vi "TDT-Get Spikes.vi"(0 "Data":T1={"TTankX"=refnum, "TDevAccX"=refnum, "LastTime"=0.0, "error"={"status"=FALSE, "code"=0, "source"=""}, "Block Name"="", "Circuit Tag"="", "Tank Name"="", "NumTicks"=0, "LastTick"=0.0, "Idle?"=FALSE, "Wait (ms)"=1000, "LastArtf"=0.0, "LastTosc"=0.0}, 7 "Max Read":i32=1000, 11 "error in (no error)":errorcluster, 13 "Tetrode":bool) -> (4 "Got 'em all":bool, 8 "Spike times":dbl[][](array[numeric]), 14 "Last Time":dbl, 15 "error out":errorcluster)   [LabVIEW 2015]
uses:
  TDT Interface Data.ctl
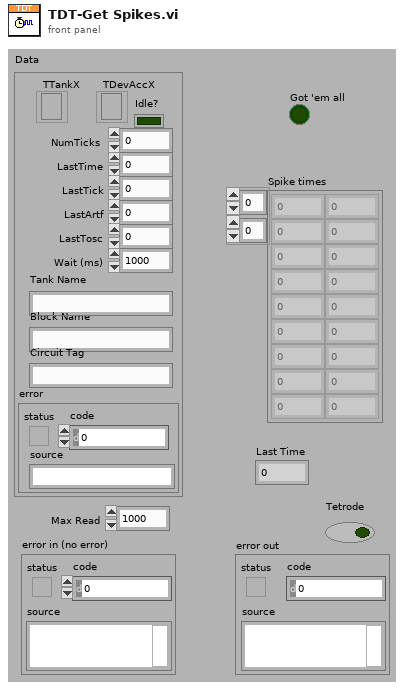
[diagram p1: front panel]
types:
  T1 = typedef "TDT Interface Data.ctl" = cluster{"TTankX":refnum<k7>, "TDevAccX":refnum<k7>, "LastTime":dbl, "error":errorcluster, "Block Name":string, "Circuit Tag":string, "Tank Name":string, "NumTicks":i32, "LastTick":dbl, "Idle?":bool, "Wait (ms)":u32, "LastArtf":dbl, "LastTosc":dbl}
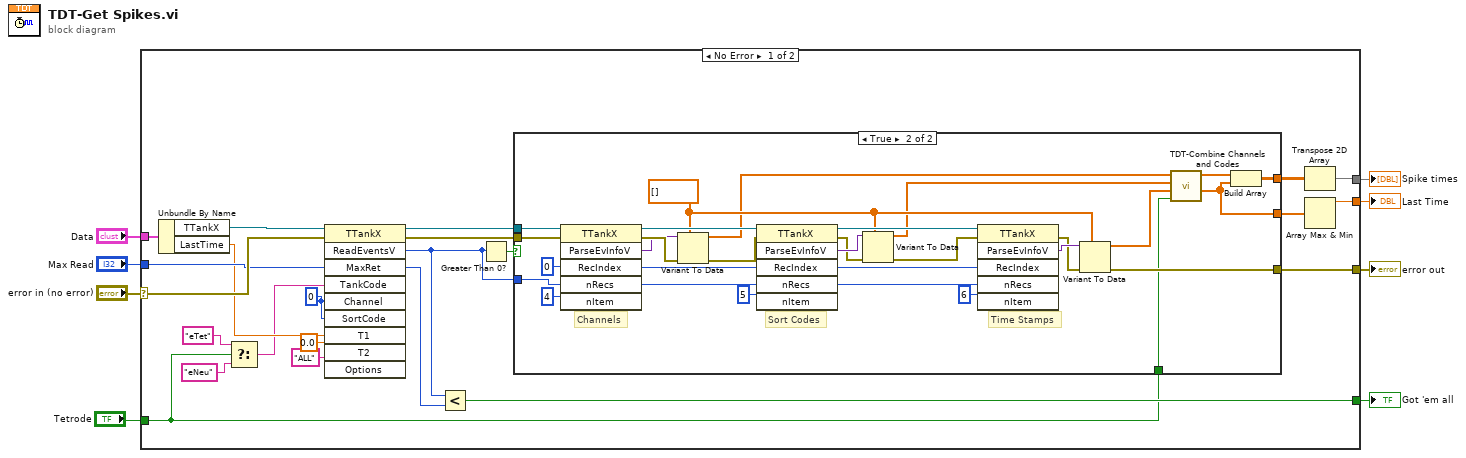
[diagram p0: block diagram]
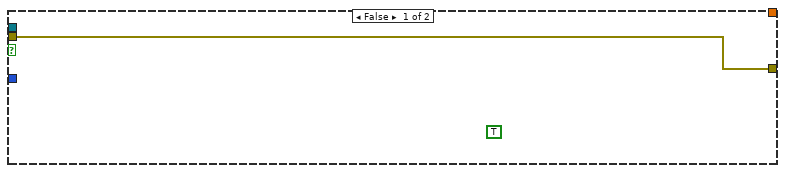
[diagram p2: hidden frame]
diagram:
  n1 = case shown="No Error" "error in (no error)" {
    selector: "error in (no error)" -> [w29 w63]
    tunnel: "Data" -> [w31 _]
    tunnel: "Max Read" -> [w28 _]
    tunnel: [w13 w63] -> w5
    tunnel: [w26 _] -> w4
    tunnel: [w15 _] -> w3
    tunnel: [w14 _] -> w2
    tunnel: "Tetrode" -> [w9 _]
    frame No Error {
      w22 = 0 ("Channel")
      n2 = Unbundle By Name(w31) -> ("TTankX"=w30:refnum<k7>, "LastTime"=w27:dbl)
      n3 = Select(t="eTet" ("TankCode"), s=w9, f="eNeu" ("TankCode")) -> (s? t:f=w10:string)
      n4 = invoke class="TTankX" method="ReadEventsV"(reference=w30, error in=w29, "MaxRet"=w28, "TankCode"=w10, "Channel"=w22, "SortCode"=w22, "T1"=w27, "T2"=0.0, "Options"="ALL") -> (reference out=w20:refnum<k7>, error out=w19:errorcluster, "ReadEventsV"=w17:i32, "MaxRet"=w21:i32)  [unwired: 1 in, 6 out]
      n5 = Less?(x=w17, y=w21) -> (x < y?=w14:bool)
      n6 = Greater Than 0?(x=w17) -> (x > 0?=w18:bool)
      n7 = case shown="True" w18 {
        tunnel: w20 -> [_ w62]
        tunnel: w19 -> [w32 w61]
        tunnel: w17 -> [_ w59]
        tunnel: [_ w36] -> w25
        tunnel: [w32 w54] -> w13
        tunnel: [_ w33] -> w16
        tunnel: w9 -> [_ w35]
        frame False {
          (unwired) TRUE
        }
        frame True {
          w41 = dbl[] []
          # "Time Stamps"
          # "Sort Codes"
          # "Channels"
          n8 = invoke class="TTankX" method="ParseEvInfoV"(reference=w62, error in=w61, "RecIndex"=0, "nRecs"=w59, "nItem"=4) -> (reference out=w51:refnum<k7>, error out=w57:errorcluster, "ParseEvInfoV"=w52:variant, "RecIndex"=w49:i32, "nRecs"=w48:i32)  [unwired: 1 in, 1 out]
          n9 = Variant To Data(error in=w57, type=w41, Variant=w52) -> (data=w39:dbl[], error out=w42:errorcluster)
          n10 = invoke class="TTankX" method="ParseEvInfoV"(reference=w51, error in=w42, "RecIndex"=w49, "nRecs"=w48, "nItem"=5) -> (reference out=w50:refnum<k7>, error out=w43:errorcluster, "ParseEvInfoV"=w44:variant, "RecIndex"=w45:i32, "nRecs"=w46:i32)  [unwired: 1 in, 1 out]
          n11 = Variant To Data(error in=w43, type=w41, Variant=w44) -> (data=w38:dbl[], error out=w37:errorcluster)
          n12 = invoke class="TTankX" method="ParseEvInfoV"(reference=w50, error in=w37, "RecIndex"=w45, "nRecs"=w46, "nItem"=6) -> (error out=w53:errorcluster, "ParseEvInfoV"=w55:variant)  [unwired: 1 in, 4 out]
          n13 = Variant To Data(error in=w53, type=w41, Variant=w55) -> (data=w34:dbl[], error out=w54:errorcluster)
          n14 = call "TDT-Combine Channels and Codes.vi"("Tetrode"=w35, "Times"=w34, "Sort Codes"=w38, "Channels"=w39) -> ("Times Out"=w33:dbl[], "Impale channel"=w40:dbl[])  [unwired: 6 in]
          n15 = Build Array(w40, w33) -> (w36:dbl[][])
        }
      }
      n16 = Transpose 2D Array(2D array=w25) -> (transposed array=w26:dbl[][])
      n17 = Array Max & Min(array=w16) -> (max value=w15:dbl)  [unwired: 3 out]
    }
    frame Error {
    }
  }
  "Spike times" <- w4
  "error out" <- w5
  "Last Time" <- w3
  "Got 'em all" <- w2
